vi "IsWarmer.vi"(10 "Alert Threshold":dbl[](array[numeric])=[4.0, 4.0, 4.0, 4.0], 11 "Temperature In":dbl[](array[numeric])=[4.0, 4.0, 4.0, 4.0]) -> (2 "String":string, 3 "Temperature is above threshold":bool)   [LabVIEW 2013]
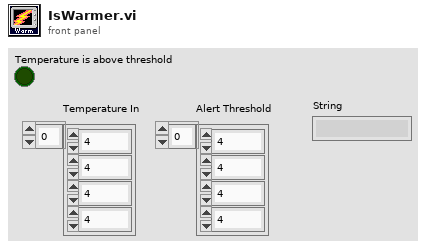
[diagram p1: front panel]
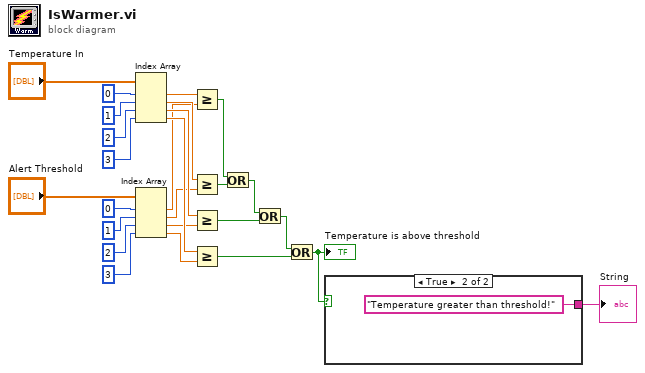
[diagram p0: block diagram]
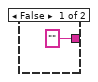
[diagram p2: hidden frame]
diagram:
  n1 = Index Array(array="Temperature In", index #1=0 ("index"), index #2=1 ("index"), index #3=2 ("index"), index #4=3 ("index")) -> (element #1=w17:dbl, element #2=w16:dbl, element #3=w15:dbl, element #4=w14:dbl)
  n2 = Index Array(array="Alert Threshold", index #1=0 ("index"), index #2=1 ("index"), index #3=2 ("index"), index #4=3 ("index")) -> (element #1=w13:dbl, element #2=w12:dbl, element #3=w11:dbl, element #4=w10:dbl)
  n3 = Greater Or Equal?(x=w17, y=w13) -> (x >= y?=w9:bool)
  n4 = Greater Or Equal?(x=w16, y=w12) -> (x >= y?=w8:bool)
  n5 = Greater Or Equal?(x=w15, y=w11) -> (x >= y?=w6:bool)
  n6 = Greater Or Equal?(x=w14, y=w10) -> (x >= y?=w4:bool)
  n7 = Or(x=w9, y=w8) -> (x .or. y?=w7:bool)
  n8 = Or(x=w7, y=w6) -> (x .or. y?=w5:bool)
  n9 = Or(x=w5, y=w4) -> (x .or. y?=w2:bool)
  "Temperature is above threshold" <- w2
  n10 = case shown="True" w2 {
    tunnel: ["" ("String") "Temperature greater than threshold!" ("String")] -> w1
    frame False {
    }
    frame True {
    }
  }
  "String" <- w1
